vi "CameraConnect.vi"(8 "error in (no error)":errorcluster, 9 "serial":u64 format="%x", 10 "name":string, 11 "CameraBase in":refnum<class "CameraBase.lvclass">) -> (0 "error out":errorcluster, 2 "CameraInfo":T1 {"serial" format="%x"}, 3 "CameraBase out":refnum<class "CameraBase.lvclass">)   [LabVIEW 2012, in "CameraBase.lvclass"]
uses:
  <userlib>/BIAS2/classes/CameraBase/CameraBase.lvclass
  <userlib>/BIAS2/classes/CameraBase/CameraInfo.ctl
  <userlib>/BIAS2/classes/CameraBase/CameraBase.lvclass/CameraBase.ctl
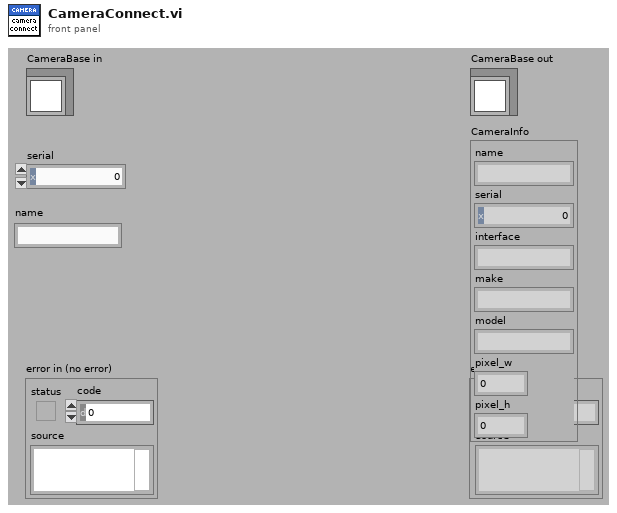
[diagram p1: front panel]
types:
  T1 = typedef "CameraInfo.ctl" = cluster{"name":string, "serial":u64, "interface":string, "make":string, "model":string, "pixel_w":dbl, "pixel_h":dbl}
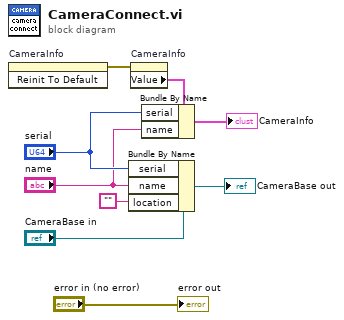
[diagram p0: block diagram]
diagram:
  n1 = invoke on="CameraInfo" class="Clust (strict)" method="Reinit To Default"() -> (error out=w4:errorcluster)  [unwired: 3 in, 2 out]
  n2 = Bundle By Name(cluster="CameraBase in", "serial"="serial", "name"="name", "location"="") -> (→"CameraBase out":refnum<class "CameraBase.lvclass">)
  n3 = property on="CameraInfo" class="Clust (strict)"(error in=w4) -> ("Value"=w2:T1)  [unwired: 1 in, 2 out]
  n4 = Bundle By Name(cluster=w2, "serial"="serial", "name"="name") -> (→"CameraInfo":T1)
  "error out" <- "error in (no error)"
